vi "Register_Value_vE.vi"(8 "error in":errorcluster, 9 "Register Value":u32, 10 "Register Number":i32, 11 "connection ID":refnum<k5>) -> (0 "error out":errorcluster, 3 "connection ID out":refnum<k5>, 5 "Match?":string, 7 "Match?":bool)   [LabVIEW 2012]
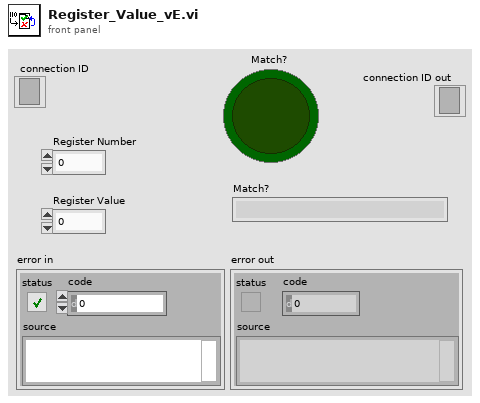
[diagram p1: front panel]
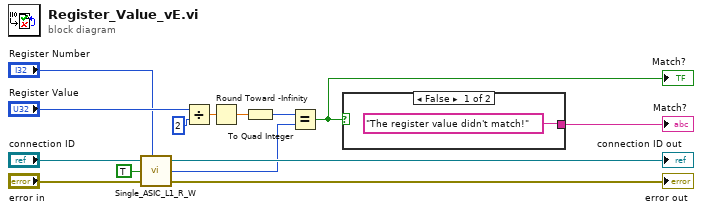
[diagram p0: block diagram]
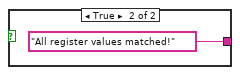
[diagram p2: hidden frame]
diagram:
  n1 = call "Single_ASIC_L1_R_W.vi"("connection ID"="connection ID", "Register or channel"="Register Number", "RD/#WR"=TRUE, "error in (no error)"="error in") -> ("connection ID out"=→"connection ID out":refnum<k5>, "data read value"=w1:i64, "error out"=→"error out":errorcluster)  [unwired: 2 in, 1 out]
  n2 = Divide(x="Register Value", y=u32 2) -> (x/y=w8:dbl)
  n3 = Round Toward -Infinity(1:w8) -> (0:w7:dbl)
  n4 = To Quad Integer(1:w7) -> (0:w10:i64)
  n5 = Equal?(x=w10, y=w1) -> (x = y?=w6:bool)
  "Match?" <- w6
  n6 = case shown="False" w6 {
    tunnel: ["The register value didn't match!" ("format string") "All register values matched!" ("format string")] -> w5
    frame False {
    }
    frame True {
    }
  }
  "Match?" <- w5
